vi "Create.vi"(8 "error in (no error)":errorcluster, 11 "obj":refnum<class "Bike.lvclass">) -> (0 "error out":errorcluster, 3 "obj out":refnum<class "Bike.lvclass">)   [LabVIEW 2019, in "Bike.lvclass"]
doc: "Creates an active by ref object.\n\nwww.sciware.com.au\nBSD License (http://www.opensource.org/licenses/bsd-license.php)"
uses:
  Bike.lvclass
  Private/DataMembers.ctl
  Bike.lvclass/Bike.ctl
panel:
  in  "data members (type)":T1
  # "BSD License (http://www.opensource.org/licenses/bsd-license.php)"
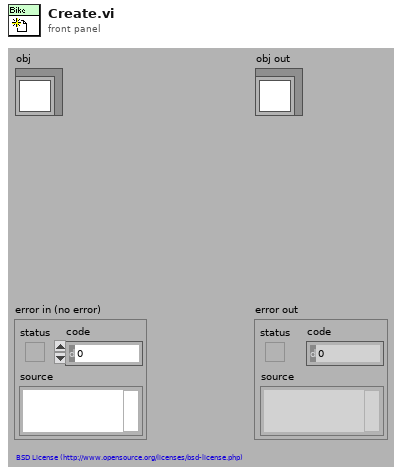
[diagram p1: front panel]
types:
  T1 = typedef "Bike.lvclass/DataMembers.ctl" = cluster{"peddle rate":dbl}
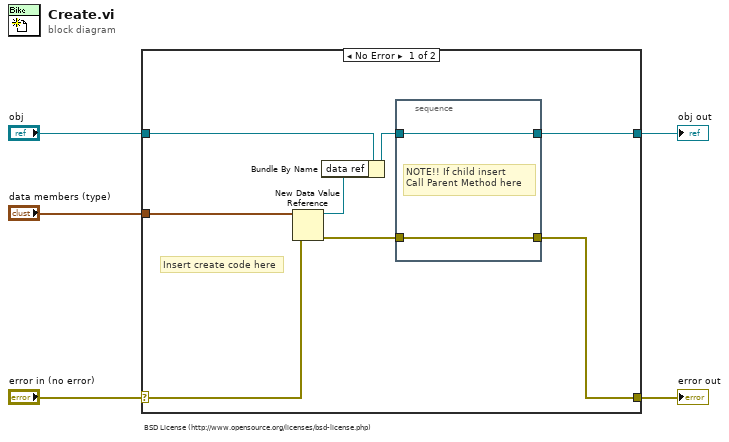
[diagram p0: block diagram]
diagram:
  # "BSD License (http://www.opensource.org/licenses/bsd-license.php)"
  n1 = case shown="No Error" "error in (no error)" {
    selector: "error in (no error)" -> [w13 w17]
    tunnel: [w6 w17] -> w4
    tunnel: "data members (type)" -> [w11 _]
    tunnel: [w7 w16] -> w2
    tunnel: "obj" -> [w10 w16]
    frame No Error {
      # "Insert create code here"
      n2 = New Data Value Reference(data value=w11, error in=w13) -> (data value reference=w12:refnum<data-value>, error out=w8:errorcluster)
      n3 = Bundle By Name(cluster=w10, "data ref"=w12) -> (w9:refnum<class "Bike.lvclass">)
      n4 = stacked-sequence {
        tunnel: [w15] -> w7
        tunnel: w9 -> [w15]
        tunnel: w8 -> [w14]
        tunnel: [w14] -> w6
        frame #0 {
          # "NOTE!! If child insert\nCall Parent Method here"
        }
      }
    }
    frame Error {
    }
  }
  "error out" <- w4
  "obj out" <- w2
